vi "StringPad.vi"(9 "width (-)":u8=2 min=2, 11 "number":i32) -> (3 "Padded string":string)   [LabVIEW 2012]
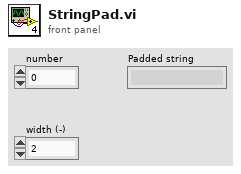
[diagram p1: front panel]
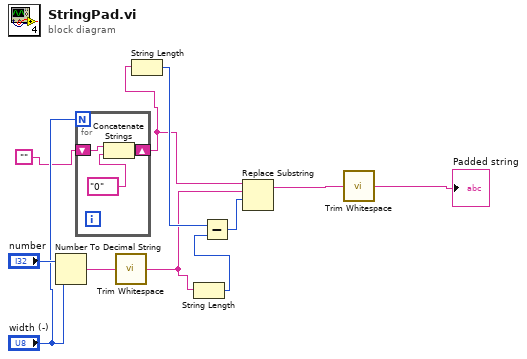
[diagram p0: block diagram]
diagram:
  n1 = Number To Decimal String(number="number", width (-)="width (-)") -> (decimal integer string=w4:string)
  n2 = for {
    N: "width (-)" -> [_]
    shift-right: [w13] -> w1
    shift-left: "" -> [w12]
    n3 = Concatenate Strings(w12, "0") -> (w13:string)
  }
  n4 = call <vilib>:"Trim Whitespace.vi"("string"=w4) -> ("trimmed string"=w5:string)  [unwired: 1 in]
  n5 = String Length(string=w1) -> (length=w11:i32)
  n6 = String Length(string=w5) -> (length=w10:i32)
  n7 = Subtract(x=w11, y=w10) -> (x-y=w9:i32)
  n8 = Replace Substring(3:w9, 4:w5, 5:w1) -> (1:w7:string)  [unwired: 1 in, 1 out]
  n9 = call <vilib>:"Trim Whitespace.vi"("string"=w7) -> ("trimmed string"=→"Padded string":string)  [unwired: 1 in]
